vi "scanner add.vi"(8 "error in":errorcluster, 10 "String":string, 11 "Config.Scanners":string[](array[string])) -> (0 "error out":errorcluster, 1 "Valid":bool, 2 "Error":string, 3 "Config.Scanners":string[](array[string]))   [LabVIEW 2023, in "User Interface.lvlib"]
uses:
  <vilib>/Utility/error.llb/Trim Whitespace One-Sided.vi
  User Interface.lvlib
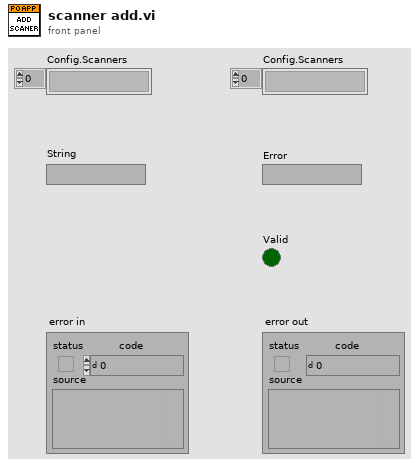
[diagram p1: front panel]
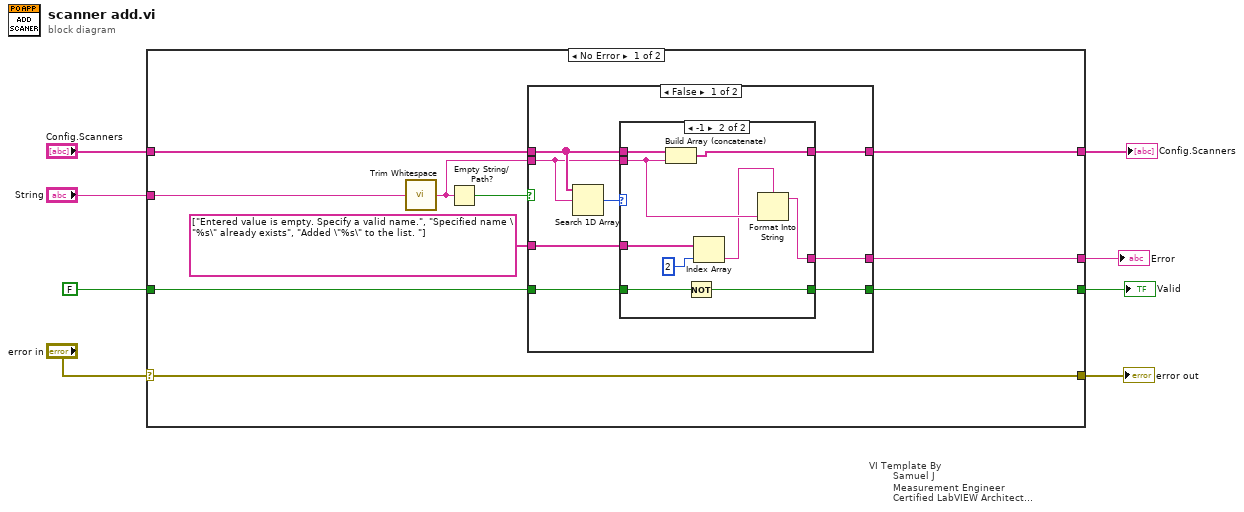
[diagram p0: block diagram]
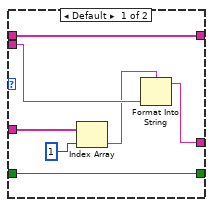
[diagram p2: hidden frame]
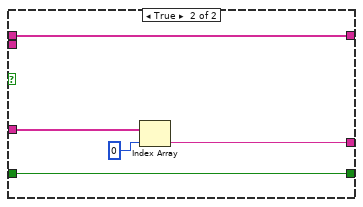
[diagram p3: hidden frame]
diagram:
  n1 = case "VI Template By\n        Samuel J\n        Measurement Engineer\n        Certified LabVIEW Architect\n        Vestas Technology R&D Chennai" shown="No Error" "error in" {
    selector: "error in" -> [w18 w50]
    tunnel: [w18 w50] -> w7
    tunnel: [w11 w49] -> w5
    tunnel: "Config.Scanners" -> [w12 w49]
    tunnel: "String" -> [w17 _]
    tunnel: [w14 w48] -> w2
    tunnel: FALSE -> [w13 w48]
    tunnel: [w9 _] -> w1
    frame No Error {
      n2 = call <vilib>:"Trim Whitespace.vi"("string"=w17) -> ("trimmed string"=w15:string)  [unwired: 1 in]
      n3 = Empty String/Path?(string/path=w15) -> (empty?=w16:bool)
      n4 = case shown="False" w16 {
        tunnel: w12 -> [w25 w47]
        tunnel: w15 -> [w24 _]
        tunnel: [w23 w47] -> w11
        tunnel: [w22 w46] -> w14
        tunnel: w13 -> [w21 w46]
        tunnel: string[] ["Entered value is empty. Specify a valid name.", "Specified name \"%s\" already exists", "Added \"%s\" to the list. "] -> [w20 w44]
        tunnel: [w19 w43] -> w9
        frame False {
          n5 = Search 1D Array(1D array=w25, element=w24) -> (index of element=w26:i32)  [unwired: 1 in]
          n6 = case shown="-1" w26 {
            tunnel: w25 -> [w33 w42]
            tunnel: w24 -> [w28 w38]
            tunnel: [w33 w41] -> w23
            tunnel: [w32 w39] -> w22
            tunnel: w21 -> [w32 w40]
            tunnel: w20 -> [w29 w36]
            tunnel: [w30 w34] -> w19
            frame Default {
              n7 = Index Array(array=w29, index=1) -> (element=w27:string)
              n8 = Format Into String(format string=w27, w28) -> (resulting string=w30:string)  [unwired: 2 in, 1 out]
            }
            frame -1 {
              n9 = Build Array (concatenate)(w42, w38) -> (w41:string[])
              n10 = Not(x=w40) -> (.not. x?=w39:bool)
              n11 = Index Array(array=w36, index=2) -> (element=w35:string)
              n12 = Format Into String(format string=w35, w38) -> (resulting string=w34:string)  [unwired: 2 in, 1 out]
            }
          }
        }
        frame True {
          n13 = Index Array(array=w44, index=0) -> (element=w43:string)
        }
      }
    }
    frame Error {
    }
  }
  "error out" <- w7
  "Config.Scanners" <- w5
  "Valid" <- w2
  "Error" <- w1
